vi "WebSocket_CreateReference.vi"(0 "ObjectReferenceToTest(Ignored If Empty)":variant, 5 "CreateMethod":T1(ring), 7 "Object name":string, 11 "error in (no error)":errorcluster) -> (4 "ObjectReferenceAsVariant":variant, 6 "NewObjectCreated":bool, 15 "error out":errorcluster)   [LabVIEW 2017, in "WebSocket.lvclass"]
doc: "This VI is used by the Debug Spawning VI, to create a DVR reference for this objects attributes."
uses:
  WebSocket.lvclass
  WebSocket.lvclass/WebSocket.ctl
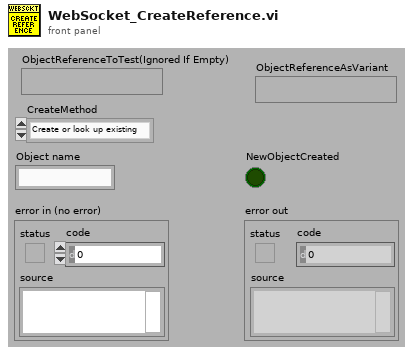
[diagram p1: front panel]
types:
  T1 = enum16{"Create or look up existing", "Look up existing"}
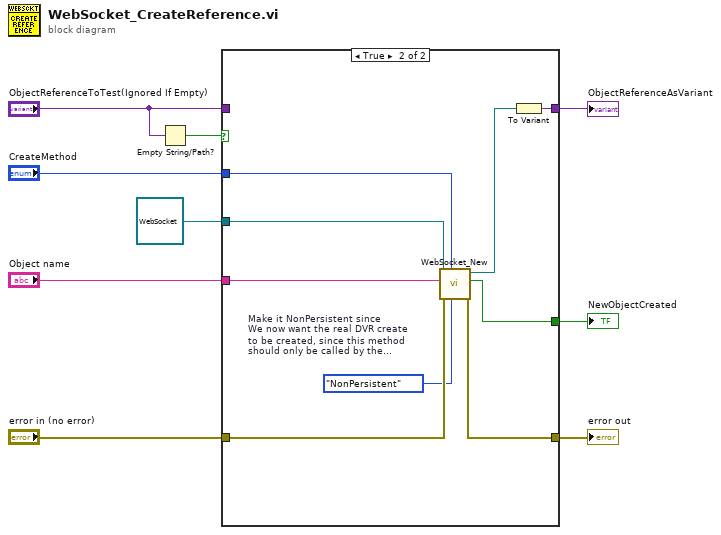
[diagram p0: block diagram]
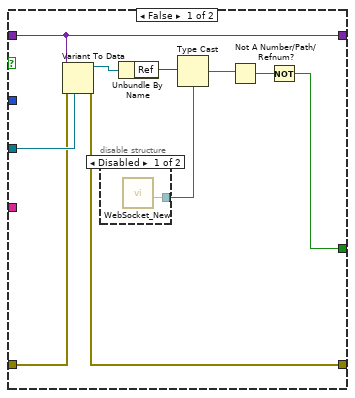
[diagram p2: hidden frame]
diagram:
  n1 = Empty String/Path?(string/path="ObjectReferenceToTest(Ignored If Empty)") -> (empty?=w3:bool)
  n2 = case shown="True" w3 {
    tunnel: "CreateMethod" -> [_ w29]
    tunnel: "error in (no error)" -> [w16 w28]
    tunnel: [w15 w27] -> w7
    tunnel: "Object name" -> [_ w26]
    tunnel: [w14 w25] -> w5
    tunnel: [w18 w23] -> w4
    tunnel: "ObjectReferenceToTest(Ignored If Empty)" -> [w18 _]
    tunnel: refnum<class "WebSocket.lvclass"> refnum ("reference in") -> [w17 w21]
    frame False {
      n3 = Variant To Data(error in=w16, type=w17, Variant=w18) -> (data=w13:refnum<class "WebSocket.lvclass">, error out=w15:errorcluster)
      n4 = disable-structure shown="Disabled" {
        disable-tunnel: [w20 _] -> w10
        frame Disabled {
          n5 = call "WebSocket_New.vi"() -> ("DVRRefOut"=w20:refnum<data-value>)  [unwired: 8 in, 3 out]
        }
        frame Enabled {
        }
      }
      n6 = Unbundle By Name(w13) -> ("Ref"=w12:u32)
      n7 = Type Cast(type=w10, x=w12) -> (*(type *) &x=w11:refnum<data-value>)
      n8 = Not A Number/Path/Refnum?(number/path/refnum=w11) -> (NaN/Path/Refnum?=w19:bool)
      n9 = Not(x=w19) -> (.not. x?=w14:bool)
    }
    frame True {
      w22 = enum16{"Default", "Persistent", "NonPersistent"}."NonPersistent"  # Make it NonPersistent since We now want the real DVR create to be created, since this method should only be called by the persistent process
      n10 = call "WebSocket_New.vi"("Persistent/Debugging(Default)"=w22, "CreateMethod(Create or look up existing)"=w29, "error in (no error)"=w28, "Object name"=w26, "reference in"=w21) -> ("error out"=w27:errorcluster, "NewObjectCreated"=w25:bool, "reference out"=w24:refnum<class "WebSocket.lvclass">)  [unwired: 3 in, 1 out]
      n11 = To Variant(anything=w24) -> (Variant=w23:variant)
    }
  }
  "error out" <- w7
  "NewObjectCreated" <- w5
  "ObjectReferenceAsVariant" <- w4
